vi "Extended Model VI.vi"(3 "output control":T1, 4 "data":variant, 5 "X":dbl[](array[numeric]), 6 "a":dbl[](array[numeric])) -> (0 "error out":errorcluster, 1 "f'(X,a)":dbl[][](array[numeric]), 2 "f(X,a)":dbl[](array[numeric]))   [LabVIEW 2022 SP3]
doc: "Implements an ellipse model function to be passed to the Nonlinear Curve Fit.vi."
uses:
  <vilib>/gmath/NumericalOptimization/LM_output select.ctl
  <vilib>/gmath/NI_Gmath.lvlib
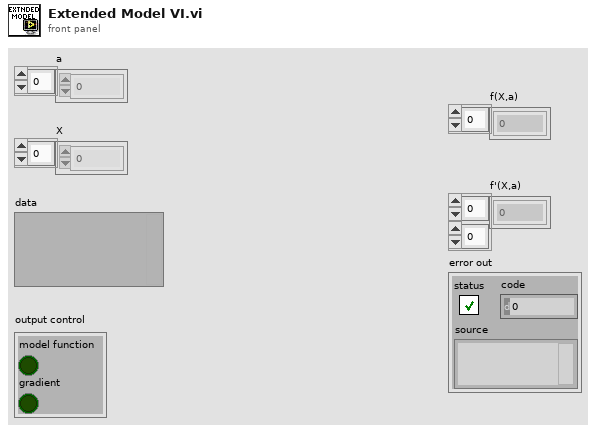
[diagram p1: front panel]
types:
  T1 = typedef "NI_Gmath.lvlib/LM_output select.ctl" = cluster{"model function":bool, "gradient":bool}
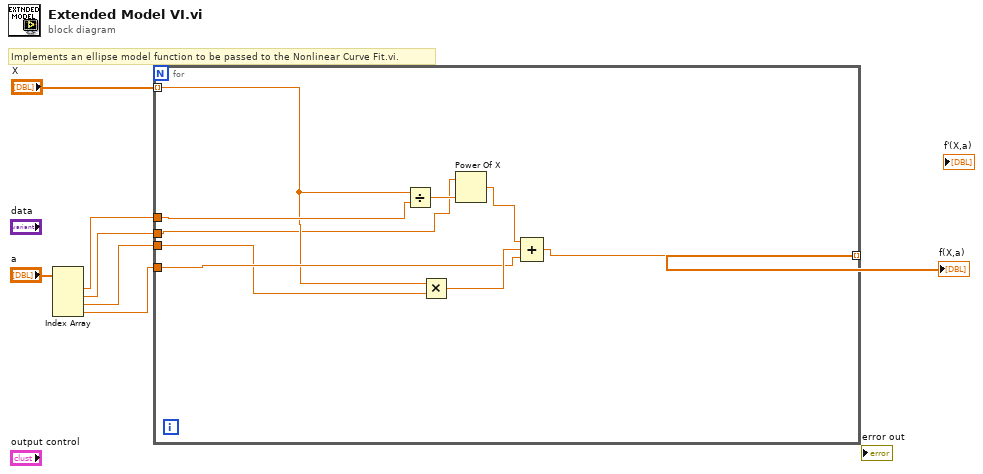
[diagram p0: block diagram]
diagram:
  # "Implements an ellipse model function to be passed to the Nonlinear Curve Fit.vi."
  n1 = Index Array(array="a") -> (element #1=w4:dbl, element #2=w3:dbl, element #3=w1:dbl, element #4=w2:dbl)  [unwired: 4 in]
  n2 = for {
    tunnel: [w11] -> w7 mode=indexing
    tunnel: "X" -> [w13] mode=indexing
    tunnel: w4 -> [w15]
    tunnel: w3 -> [w9]
    tunnel: w2 -> [w14]
    tunnel: w1 -> [w12]
    n3 = Divide(x=w13, y=w15) -> (x/y=w10:dbl)
    n4 = Multiply(x=w13, y=w12) -> (x*y=w16:dbl)
    n5 = Power Of X(1:w10, 2:w9) -> (0:w8:dbl)
    n6 = Compound Arithmetic op=ADD(w8, w16, w14) -> (w11:dbl)
  }
  "f(X,a)" <- w7
